vi "Channel Status.vi"(5 "All Channels (T)":bool=TRUE, 7 "Channel":u8, 8 "error in (no error)":errorcluster, 11 "BoardHandle":T2) -> (0 "error out":errorcluster, 1 "Channel Status (decimal value)":i32[](array[numeric]), 2 "Channel Status Array":T1(array[cluster]), 3 "BoardHandle out":T2)   [LabVIEW 2020, in "CAEN PSM.lvlib"]
doc: "Returns status for channels or a desired channel."
uses:
  CAEN PSM.lvlib
  BoardHandle.ctl
panel:
  # "The meaning of the bits may differ\ndepending on the device model"
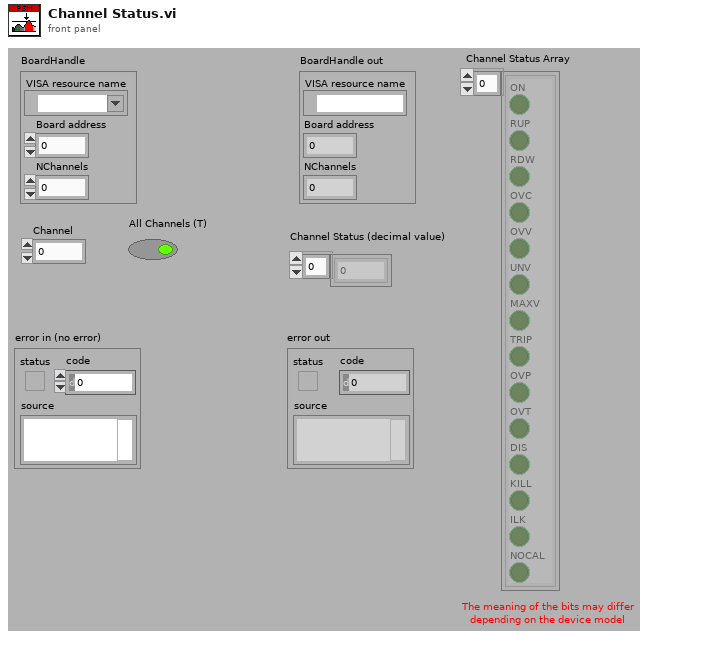
[diagram p1: front panel]
types:
  T1 = cluster{"ON":bool, "RUP":bool, "RDW":bool, "OVC":bool, "OVV":bool, "UNV":bool, "MAXV":bool, "TRIP":bool, "OVP":bool, "OVT":bool, "DIS":bool, "KILL":bool, "ILK":bool, "NOCAL":bool}[]
  T2 = typedef "CAEN PSM.lvlib/BoardHandle.ctl" = cluster{"VISA resource name":refnum<visa-resource-name>, "Board address":i8, "NChannels":u8}
  T3 = cluster{"OVV":bool, "UNV":bool, "MAXV":bool, "TRIP":bool, "OVP":bool, "OVT":bool, "DIS":bool, "KILL":bool, "ILK":bool, "OVC":bool, "RDW":bool, "RUP":bool, "ON":bool, "NOCAL":bool}[]
  T4 = cluster{"Boolean array[0]":bool, "Boolean array[1]":bool, "Boolean array[2]":bool, "Boolean array[3]":bool, "Boolean array[4]":bool, "Boolean array[5]":bool, "Boolean array[6]":bool, "Boolean array[7]":bool, "Boolean array[8]":bool, "Boolean array[9]":bool, "Boolean array[10]":bool, "Boolean array[11]":bool, "Boolean array[12]":bool, "Boolean array[13]":bool}
  T5 = cluster{"Boolean array[0]":bool, "Boolean array[1]":bool, "Boolean array[2]":bool, "Boolean array[3]":bool, "Boolean array[4]":bool, "Boolean array[5]":bool, "Boolean array[6]":bool, "Boolean array[7]":bool, "Boolean array[8]":bool, "Boolean array[9]":bool, "Boolean array[10]":bool, "Boolean array[11]":bool, "Boolean array[12]":bool, "Boolean array[13]":bool}[]
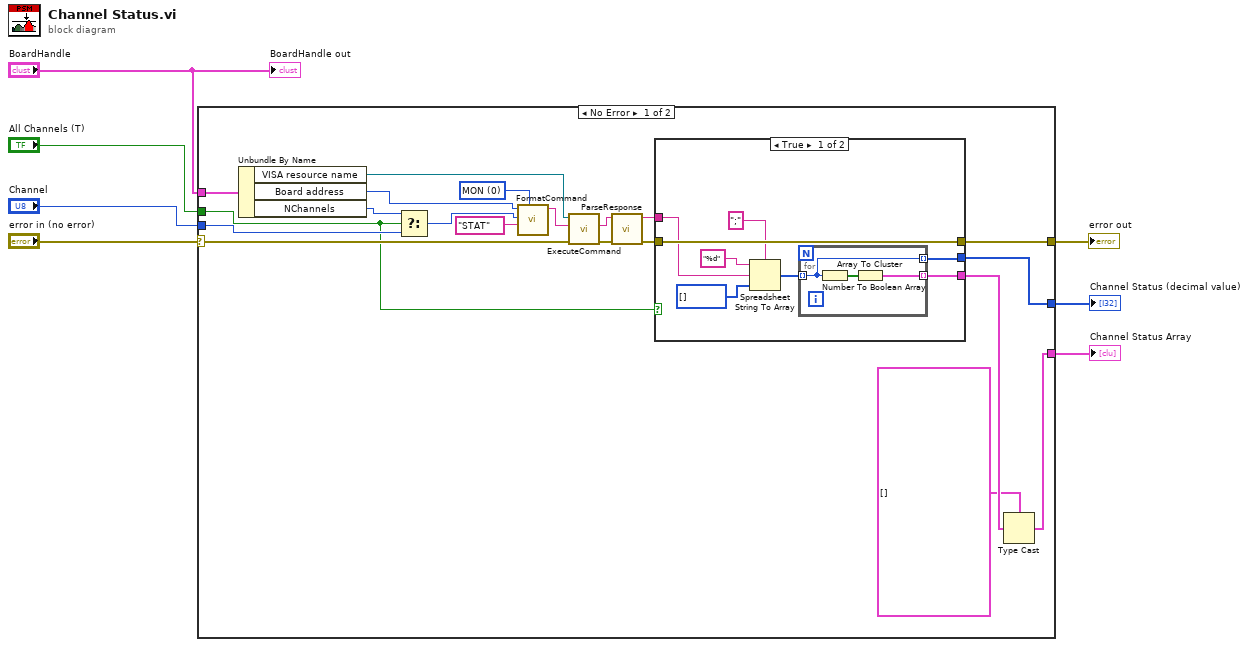
[diagram p0: block diagram]
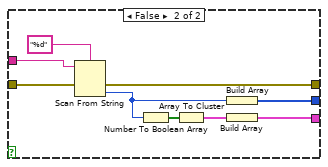
[diagram p2: hidden frame]
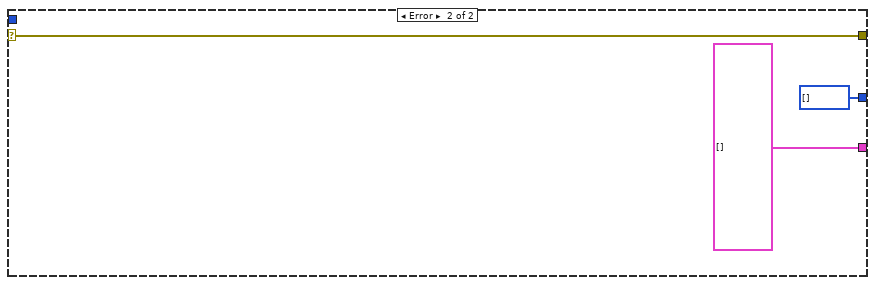
[diagram p3: hidden frame]
diagram:
  n1 = case shown="No Error" "error in (no error)" {
    selector: "error in (no error)" -> [w18 w50]
    tunnel: "All Channels (T)" -> [w9 _]
    tunnel: "Channel" -> [w25 _]
    tunnel: [w10 w50] -> w4
    tunnel: "BoardHandle" -> [w19 _]
    tunnel: [w11 T3 []] -> w2
    tunnel: [w8 i32[] []] -> w1
    frame No Error {
      w26 = u8 0 items=["MON", "SET"] ("CMD")
      n2 = Unbundle By Name(w19) -> ("VISA resource name"=w23:refnum<visa-resource-name>, "Board address"=w27:i8, "NChannels"=w15:u8)
      n3 = Select(t=w15, s=w9, f=w25) -> (s? t:f=w24:u8)
      n4 = call "FormatCommand.vi"("CMD (MON)"=w26, "PAR"="STAT", "CH"=w24, "BD (0)"=w27) -> ("cmd"=w22:string)  [unwired: 7 in]
      n5 = call "ExecuteCommand.vi"("error in (no error)"=w18, "Command"=w22, "VISA resource name"=w23) -> ("error out"=w21:errorcluster, "Response"=w20:string)  [unwired: 6 in, 1 out]
      n6 = call "ParseResponse.vi"("error in (no error)"=w21, "Response"=w20) -> ("error out"=w14:errorcluster, "val"=w16:string)  [unwired: 6 in, 2 out]
      n7 = case shown="True" w9 {
        tunnel: w16 -> [w33 w47]
        tunnel: w14 -> [w35 w45]
        tunnel: [w29 w42] -> w13
        tunnel: [w35 w44] -> w10
        tunnel: [w28 w39] -> w8
        frame True {
          n8 = Spreadsheet String To Array(delimiter (Tab)=";", format string="%d", spreadsheet string=w33, array type (2D Dbl)=i32[] []) -> (array=w30:i32[])
          n9 = for {
            tunnel: w30 -> [w36] mode=indexing
            tunnel: [w38] -> w29 mode=indexing
            tunnel: [w36] -> w28 mode=indexing
            n10 = Number To Boolean Array(number=w36) -> (Boolean array=w37:bool[])
            n11 = Array To Cluster(array=w37) -> (cluster=w38:T4)
          }
        }
        frame False {
          n12 = Scan From String(format string="%d", input string=w47, error in=w45) -> (error out=w44:errorcluster, output 1=w40:i32)  [unwired: 2 in, 2 out]
          n13 = Number To Boolean Array(number=w40) -> (Boolean array=w41:bool[])
          n14 = Array To Cluster(array=w41) -> (cluster=w43:T4)
          n15 = Build Array(w40) -> (w39:i32[])
          n16 = Build Array(w43) -> (w42:T5)
        }
      }
      n17 = Type Cast(type=T1 [], x=w13) -> (*(type *) &x=w11:T1)
    }
    frame Error {
    }
  }
  "error out" <- w4
  "Channel Status Array" <- w2
  "Channel Status (decimal value)" <- w1
  "BoardHandle out" <- "BoardHandle"
